vi "Read Configuration.vi"(8 "error in (no error)":errorcluster) -> (0 "error out":errorcluster, 2 "Switch Schedule Out":T1)   [LabVIEW 2014]
uses:
  Controls/Switch Schedule.ctl
  Controls/Switch Program.ctl
  Controls/Action Enum.ctl
  Controls/Switch Day.ctl
  <vilib>/Utility/config.llb/Read Key (String).vi
  <vilib>/Utility/config.llb/NI_LVConfig.lvlib
panel:
  in  "Switch Schedule":T1
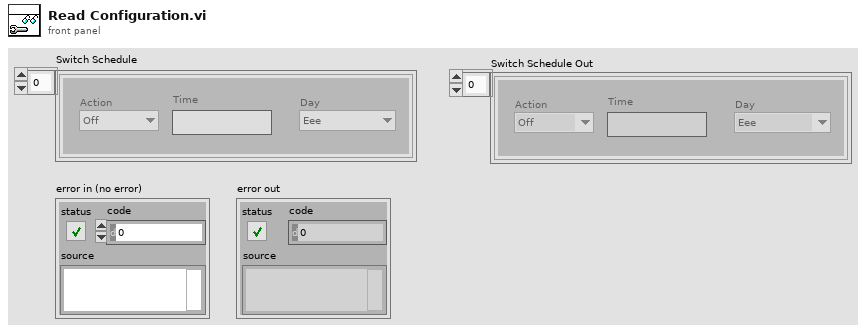
[diagram p1: front panel]
types:
  T1 = typedef "Switch Schedule.ctl" = T2[]
  T2 = typedef "Switch Program.ctl" = cluster{"Action":T3, "Time":string, "Day":T4}
  T3 = typedef "Action Enum.ctl" = enum16{"Off", "On"}
  T4 = typedef "Switch Day.ctl" = enum16{"Eee", "Sun", "Mon", "Tue", "Wed", "Thu", "Fri", "Sat"}
  T5 = typedef "NI_LVConfig.lvlib/Config Data RefNum.ctl" = refnum<k1>
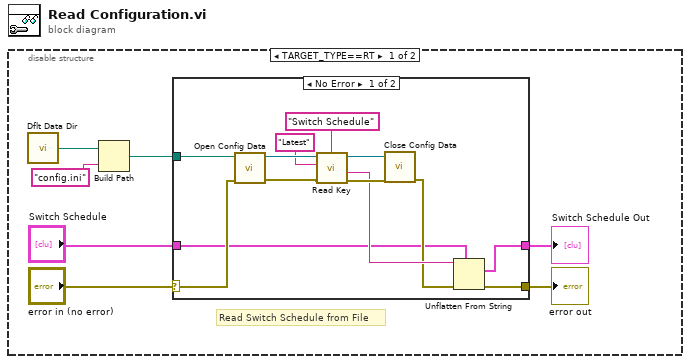
[diagram p0: block diagram]
diagram:
  n1 = disable-structure shown="TARGET_TYPE==RT" {
    frame condition #0 (active) {
      # "Read Switch Schedule from File"
      n2 = call <vilib>:"Dflt Data Dir.vi"() -> ("App:Default Data Directory"=w7:path)
      n3 = Build Path(base path=w7, name or relative path="config.ini") -> (appended path=w5:path)
      n4 = case shown="No Error" "error in (no error)" {
        selector: "error in (no error)" -> [w13 w22]
        tunnel: w5 -> [w20 _]
        tunnel: "Switch Schedule" -> [w9 w21]
        tunnel: [w10 w22] -> w2
        tunnel: [w8 w21] -> w1
        frame No Error {
          n5 = call <vilib>:"Open Config Data.vi"("error in (no error)"=w13, "configuration file path"=w20) -> ("error out"=w18:errorcluster, "refnum"=w19:T5)  [unwired: 7 in, 1 out]
          n6 = call-poly <vilib>:"Read Key.vi"("section"="Switch Schedule", "error in (no error)"=w18, "key"="Latest", "refnum"=w19) -> ("error out"=w14:errorcluster, "value"=w12:string, "refnum out"=w15:T5)  [unwired: 4 in, 1 out]
          n7 = call <vilib>:"Close Config Data.vi"("error in (no error)"=w14, "refnum"=w15) -> ("error out"=w11:errorcluster)  [unwired: 8 in, 1 out]
          n8 = Unflatten From String(type=w9, binary string=w12, error in (no error)=w11) -> (value=w8:T1, error out=w10:errorcluster)  [unwired: 2 in, 1 out]
        }
        frame Error {
        }
      }
      "error out" <- w2
      "Switch Schedule Out" <- w1
    }
    frame condition #1 {
    }
  }
